vi "Configure sub-VI.vi"(8 "error in":errorcluster, 9 "Update Config":bool, 10 "Port Configurations":T6(array[cluster]), 11 "FPGA VI Reference In":refnum<k20>) -> (0 "error out":errorcluster, 3 "FPGA VI Reference Out":refnum<k20>)   [LabVIEW 2010]
doc: "Configures all serial ports in the system. This VI takes an array of the Port Configuration Cluster Control (Serial Port Parameters.ctl located under the cRIO target in the project) and sends the values to the FPGA VI via a Read/Write Control.\n\nThis subVI is designed to shrink and grow with the number of serial ports which need to be controled. Simply add or remove elements from/to the Read/Write Control in the True Case of the Case Structure."
uses:
  <vilib>/LabVIEW Targets/FPGA/cRIO/shared/nicrio_ModuleControls/nicrio_cRIO-9871_BaudRateEnum.ctl
  <vilib>/LabVIEW Targets/FPGA/cRIO/shared/nicrio_ModuleControls/nicrio_cRIO-9871_DataBitsEnum.ctl
  <vilib>/LabVIEW Targets/FPGA/cRIO/shared/nicrio_ModuleControls/nicrio_cRIO-9871_ParityEnum.ctl
  <vilib>/LabVIEW Targets/FPGA/cRIO/shared/nicrio_ModuleControls/nicrio_cRIO-9871_StopBitsEnum.ctl
  <vilib>/LabVIEW Targets/FPGA/cRIO/shared/nicrio_ModuleControls/nicrio_cRIO-9871_FlowControlEnum.ctl
  <vilib>/rvi/interface/nirviReadWriteControl/nirviReadWriteControl.xnode
  <vilib>/rvi/interface/common/niFpgaNodeNameForErrorReporting.ctl
  <vilib>/rvi/errors/niLvFpgaWhatHappensToTopLevelVI.ctl
  <vilib>/Utility/error.llb/Error Cluster From Error Code.vi
  <vilib>/rvi/errors/niLvFpgaAdjustHostInterfaceError.vi
  NiFpgaLv.dll
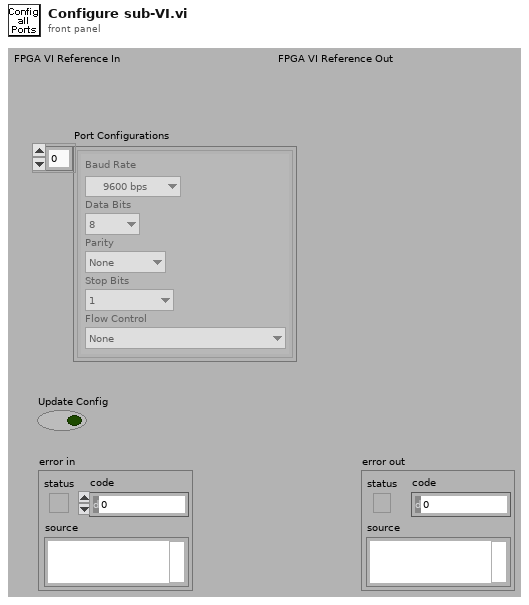
[diagram p1: front panel]
types:
  T1 = typedef "nicrio_cRIO-9871_BaudRateEnum.ctl" = enum16{"75 bps", "110 bps", "134 bps", "150 bps", "300 bps", "600 bps", "1200 bps", "1800 bps", "2400 bps", "4800 bps", "7200 bps", "9600 bps", "14.4 kbps", "19.2 kbps", "28.8 kbps", "38.4 kbps", "57.6 kbps", "115.2 kbps", "230.4 kbps", "460.8 kbps", "921.6 kbps"}
  T2 = typedef "nicrio_cRIO-9871_DataBitsEnum.ctl" = enum8{"5", "6", "7", "8"}
  T3 = typedef "nicrio_cRIO-9871_ParityEnum.ctl" = enum8{"None", "Odd", "Even", "Mark", "Space"}
  T4 = typedef "nicrio_cRIO-9871_StopBitsEnum.ctl" = enum8{"1", "1.5", "2"}
  T5 = typedef "nicrio_cRIO-9871_FlowControlEnum.ctl" = enum8{"None", "Software (XON / XOFF)", "Hardware (RTS / CTS)"}
  T6 = cluster{"Baud Rate":T1, "Data Bits":T2, "Parity":T3, "Stop Bits":T4, "Flow Control":T5}[]
  T7 = typedef "niFpgaNodeNameForErrorReporting.ctl" = enum16{"Open FPGA VI Reference", "Read/Write Control", "Invoke Method: Abort", "Invoke Method: Acknowledge IRQ", "Invoke Method: Download", "Invoke Method: FIFO.Configure", "Invoke Method: FIFO.Read", "Invoke Method: FIFO.Start", "Invoke Method: FIFO.Stop", "Invoke Method: FIFO.Write", "Invoke Method: Reset", "Invoke Method: Run", "Invoke Method: Wait on IRQ", "Close FPGA VI Reference"}
  T8 = typedef "niLvFpgaWhatHappensToTopLevelVI.ctl" = enum16{"top level VI scripted behind XNode", "top level VI inlined behind XNode"}
  T9 = cluster{"Baud Rate":T1, "Data Bits":T2, "Parity":T3, "Stop Bits":T4, "Flow Control":T5}
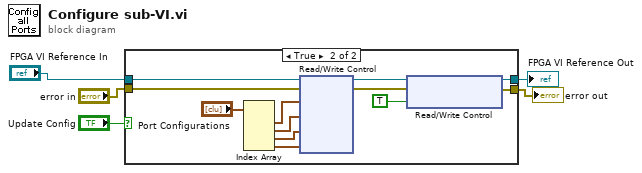
[diagram p0: block diagram]
diagram:
  n1 = case shown="True" "Update Config" {
    tunnel: "error in" -> [w7 w19]
    tunnel: "FPGA VI Reference In" -> [w6 w18]
    tunnel: [w7 w16] -> w4
    tunnel: [w6 w17] -> w1
    frame False {
    }
    frame True {
      n2 = Index Array(array="Port Configurations") -> (element #1=w11:T9, element #2=w10:T9, element #3=w9:T9, element #4=w8:T9)  [unwired: 4 in]
      n3 = xnode "Read/Write Control"("FPGA VI Reference In"=w18, "error in"=w19, "Port 1"=w11, "Port 2"=w10, "Port 3"=w9, "Port 4"=w8) -> ("FPGA VI Reference Out"=w13:refnum<k20>, "error out"=w14:errorcluster)
      n4 = xnode "Read/Write Control"("FPGA VI Reference In"=w13, "error in"=w14, "Update Config"=TRUE) -> ("FPGA VI Reference Out"=w17:refnum<k20>, "error out"=w16:errorcluster)
    }
  }
  "error out" <- w4
  "FPGA VI Reference Out" <- w1
